vi "Process Pulse.vi"(8 "error in (no error)":errorcluster, 10 "Input":T2={"From"="broadcaster", "To"="broadcaster", "Pulse"=FALSE}, 11 "Conjunction in":refnum<class "Conjunction.lvclass">) -> (0 "error out":errorcluster, 2 "Outputs":T1(array[cluster]), 3 "Conjunction out":refnum<class "Conjunction.lvclass">)   [LabVIEW 2021, in "Conjunction.lvclass"]
uses:
  Conjunction.lvclass
  Conjunction.lvclass/Conjunction.ctl
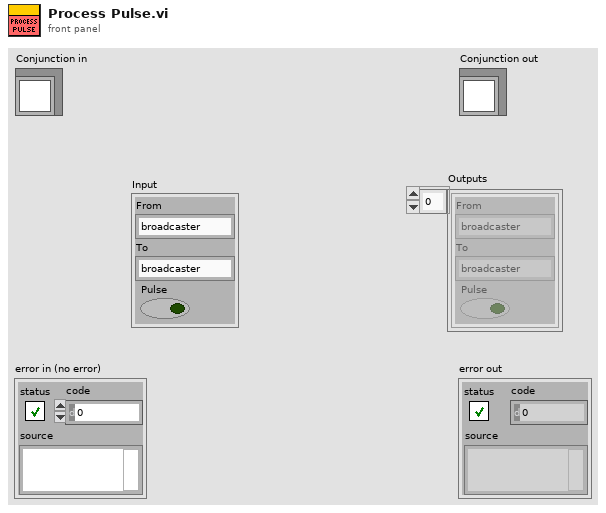
[diagram p1: front panel]
types:
  T1 = cluster{"From":string, "To":string, "Pulse":bool}[]
  T2 = cluster{"From":string, "To":string, "Pulse":bool}
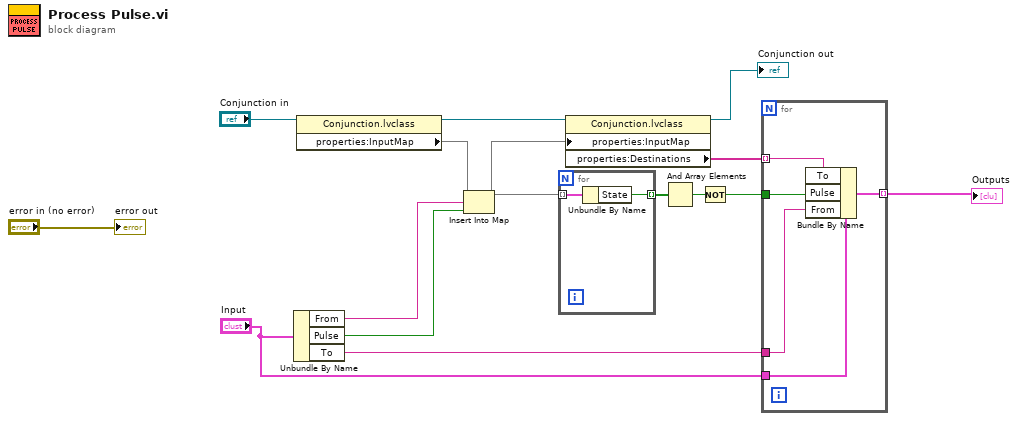
[diagram p0: block diagram]
diagram:
  n1 = Unbundle By Name("Input") -> ("From"=w12:string, "Pulse"=w11:bool, "To"=w3:string)
  n2 = property class="Conjunction.lvclass"(reference="Conjunction in") -> (reference out=w10:refnum<class "Conjunction.lvclass">, "properties:InputMap"=w13:map{string, bool})  [unwired: 1 in, 1 out]
  n3 = Insert Into Map(map in=w13, key=w12, value=w11) -> (map out=w9:map{string, bool})  [unwired: 2 out]
  n4 = for {
    tunnel: w9 -> [w17] mode=indexing
    tunnel: [w16] -> w8 mode=indexing
    n5 = Unbundle By Name(w17) -> ("State"=w16:bool)
  }
  n6 = property class="Conjunction.lvclass"(reference=w10, "properties:InputMap"=w9) -> (reference out=→"Conjunction out":refnum<class "Conjunction.lvclass">, "properties:Destinations"=w5:string[])  [unwired: 1 in, 1 out]
  n7 = And Array Elements(Boolean array=w8) -> (logical AND=w7:bool)
  n8 = Not(x=w7) -> (.not. x?=w4:bool)
  n9 = for {
    tunnel: w5 -> [w19] mode=indexing
    tunnel: w4 -> [w20]
    tunnel: w3 -> [w21]
    tunnel: "Input" -> [w22]
    tunnel: [w18] -> w1 mode=indexing
    n10 = Bundle By Name(cluster=w22, "To"=w19, "Pulse"=w20, "From"=w21) -> (w18:T2)
  }
  "Outputs" <- w1
  "error out" <- "error in (no error)"
